vi "Open Sequence File.vi"(8 "error in":errorcluster) -> (0 "error out":errorcluster, 2 "Valid?":bool, 3 "Configured Steps Out":T1[](array[typedef]))   [LabVIEW 2018]
doc: "Open the control sequence file (a datalog file) and verifies that the sequence is compatible with the current version of the LabVIEW Real-Time Sequencer."
uses:
  controls/Configured Step.ctl
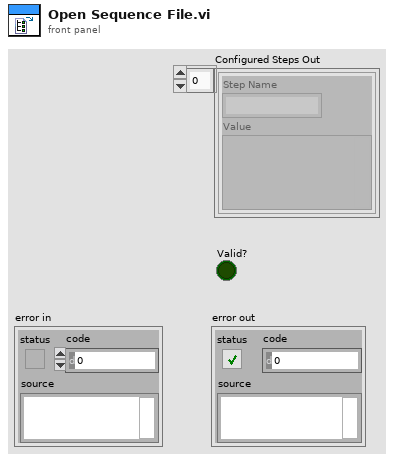
[diagram p1: front panel]
types:
  T1 = typedef "Configured Step.ctl" = cluster{"Step Name":string, "Value":variant}
  T2 = enum16{"open", "replace", "create", "open or create", "replace or create", "replace or create with confirmation"}
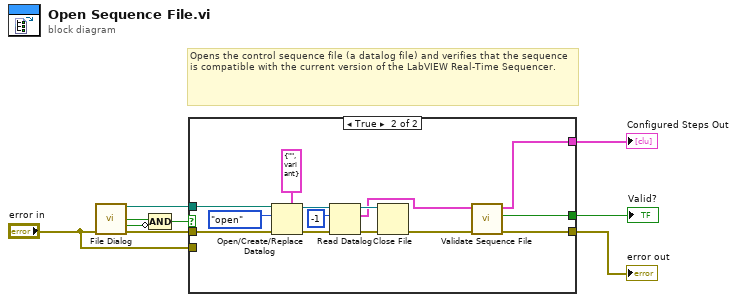
[diagram p0: block diagram]
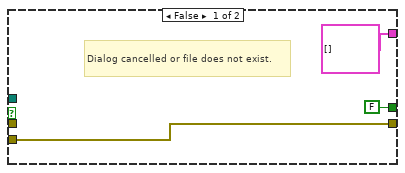
[diagram p2: hidden frame]
diagram:
  # "Opens the control sequence file (a datalog file) and verifies that the sequence is compatible with the current version of the LabVIEW Real-Time Sequencer."
  n1 = call "File Dialog"("error in"="error in") -> ("selected path"=w6:path, "exists"=w9:bool, "cancelled"=w8:bool, "error out"=w5:errorcluster)  [unwired: 11 in]
  n2 = Compound Arithmetic op=AND(w9, invert w8) -> (w7:bool)
  n3 = case shown="True" w7 {
    tunnel: [T1[] [] w14] -> w4
    tunnel: [w10 w16] -> w3
    tunnel: w6 -> [_ w19]
    tunnel: w5 -> [_ w18]
    tunnel: [FALSE ("Valid?") w13] -> w2
    tunnel: "error in" -> [w10 _]
    frame False {
      # "Dialog cancelled or file does not exist."
    }
    frame True {
      n4 = Open/Create/Replace Datalog(5:T1 {"Step Name"="", "Value"=variant} ("Configured Step"), 8:w18, 10:T2."open" ("operation (0:open)"), 11:w19) -> (0:w26:errorcluster, 3:w21:refnum<k1>)  [unwired: 2 in, 1 out]
      n5 = Read Datalog(4:w26, 6:-1 ("count (1)"), 7:w21) -> (0:w24:errorcluster, 2:w15:T1[], 3:w23:refnum<k1>)
      n6 = Close File(refnum=w23, error in=w24) -> (error out=w17:errorcluster)  [unwired: 1 out]
      n7 = call "Validate Sequence File.vi"("error in (no error)"=w17, "Configured Steps In"=w15) -> ("error out"=w16:errorcluster, "Valid?"=w13:bool, "Configured Steps Out"=w14:T1[])  [unwired: 7 in]
    }
  }
  "Configured Steps Out" <- w4
  "error out" <- w3
  "Valid?" <- w2
